vi "initialiseDevice.vi"(8 "error in (no error)":errorcluster, 10 "deviceName":string, 11 "BECHWCBasic in":refnum<class "BECHWCBasic.lvclass">) -> (0 "error out":errorcluster, 3 "BECHWCBasic out":refnum<class "BECHWCBasic.lvclass">)   [LabVIEW 2011, in "Hardware.lvlib" / "HWControllers.lvlib" / "BECHWCBasic.lvclass"]
doc: "Initialise a hardware device. \nI.e. set its initial channel states etc."
uses:
  BECHWCBasic.lvclass
  BECHWCBasic.lvclass/BECHWCBasic.ctl
  Channels/VoltOutput/AnalogOutput.lvclass
  Channels/Digital/DigitalOutput.lvclass
  HWController.lvclass
  Tools/DatabaseHelpers/DbConnection/DeviceDataBase/deviceDataBase.lvclass
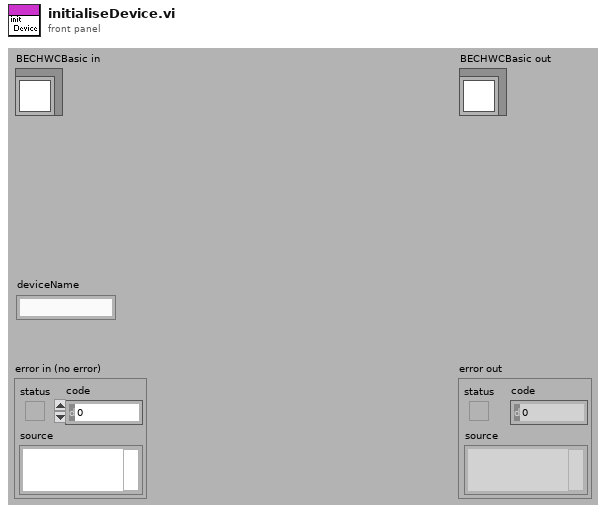
[diagram p1: front panel]
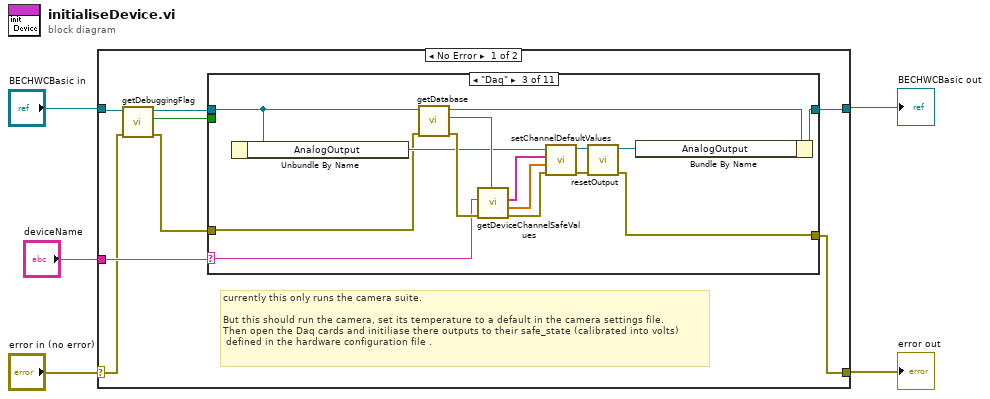
[diagram p0: block diagram]
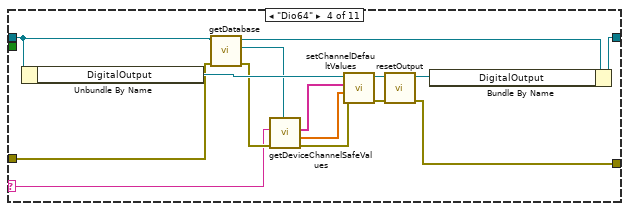
[diagram p4: hidden frame]
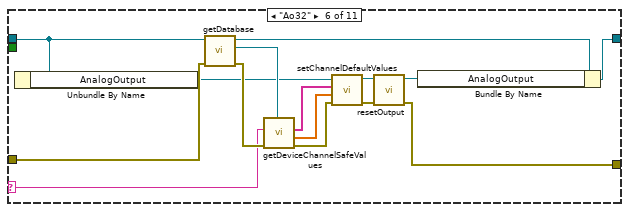
[diagram p6: hidden frame]
diagram:
  n1 = case shown="No Error" "error in (no error)" {
    selector: "error in (no error)" -> [w8 w76]
    tunnel: [w11 w76] -> w4
    tunnel: [w13 w75] -> w2
    tunnel: "BECHWCBasic in" -> [w10 w75]
    tunnel: "deviceName" -> [w12 _]
    frame No Error {
      # "currently this only runs the camera suite. \n\nBut this should run the camera, set its temperature to a default in the camera settings file.\nThen open the Daq cards and initiliase there outputs to their safe_state (calibrated into volts)\n defined in the hardware configuration file ."
      n2 = call "getDebuggingFlag.vi"("error in (no error)"=w8, "HWController.lvclass in"=w10) -> ("error out"=w7:errorcluster, "debuggingFlag"=w6:bool, "HWController.lvclass out"=w9:refnum<class "BECHWCBasic.lvclass">)  [unwired: 7 in]
      n3 = case shown="\"Daq\"" w12 {
        selector: w12 -> [_ _ w18 w37 _ w62 _ _ _ _ _]
        tunnel: w9 -> [w15 w17 w22 w41 w48 w55 w66 w68 w70 w72 w74]
        tunnel: [w15 w17 w19 w43 w48 w50 w66 w68 w70 w72 w74] -> w13
        tunnel: w7 -> [w14 w16 w21 w33 w49 w61 w65 w67 w69 w71 w73]
        tunnel: [w14 w16 w20 w42 w49 w53 w65 w67 w69 w71 w73] -> w11
        tunnel: w6 -> [_ _ _ _ _ _ _ _ _ _ _]
        frame "No Hardware", Default {
        }
        frame "UsbDAQ" {
        }
        frame "Daq" {
          n4 = Unbundle By Name(w22) -> ("AnalogOutput"=w25:refnum<class "AnalogOutput.lvclass">)
          n5 = call "getDatabase.vi"("error in (no error)"=w21, "HWController in"=w22) -> ("error out"=w31:errorcluster, "deviceDataBase"=w32:refnum<class "deviceDataBase.lvclass">, "HWController out"=w23:refnum<class "BECHWCBasic.lvclass">)  [unwired: 7 in]
          n6 = call "getDeviceChannelSafeValues.vi"("error in (no error)"=w31, "device_name"=w18, "deviceDataBase in"=w32) -> ("error out"=w30:errorcluster, "SafeVaues"=w29:dbl[], "ChannelAddresses"=w28:string[])  [unwired: 5 in, 1 out]
          n7 = call "setChannelDefaultValues.vi"("error in (no error)"=w30, "calibratedValues"=w29, "channel_addresses"=w28, "AnalogOutput in"=w25) -> ("error out"=w26:errorcluster, "AnalogOutput out"=w27:refnum<class "AnalogOutput.lvclass">)  [unwired: 6 in]
          n8 = call-dynamic "resetOutput.vi"("error in (no error)"=w26, "AnalogOutput in"=w27) -> ("error out"=w20:errorcluster, "AnalogOutput out"=w24:refnum<class "AnalogOutput.lvclass">)  [unwired: 8 in]
          n9 = Bundle By Name(cluster=w23, "AnalogOutput"=w24) -> (w19:refnum<class "BECHWCBasic.lvclass">)
        }
        frame "Dio64" {
          n10 = Unbundle By Name(w41) -> ("DigitalOutput"=w47:refnum<class "DigitalOutput.lvclass">)
          n11 = call "getDatabase.vi"("error in (no error)"=w33, "HWController in"=w41) -> ("error out"=w38:errorcluster, "deviceDataBase"=w39:refnum<class "deviceDataBase.lvclass">, "HWController out"=w40:refnum<class "BECHWCBasic.lvclass">)  [unwired: 7 in]
          n12 = call "getDeviceChannelSafeValues.vi"("error in (no error)"=w38, "device_name"=w37, "deviceDataBase in"=w39) -> ("error out"=w34:errorcluster, "SafeVaues"=w35:dbl[], "ChannelAddresses"=w36:string[])  [unwired: 5 in, 1 out]
          n13 = call-dynamic "setChannelDefaultValues.vi"("error in (no error)"=w34, "calibratedValues"=w35, "channel_addresses"=w36, "DigitalOutput in"=w47) -> ("error out"=w45:errorcluster, "DigitalOutput out"=w46:refnum<class "DigitalOutput.lvclass">)  [unwired: 6 in]
          n14 = call-dynamic "resetOutput.vi"("error in (no error)"=w45, "DigitalOutput in"=w46) -> ("error out"=w42:errorcluster, "DigitalOutput out"=w44:refnum<class "DigitalOutput.lvclass">)  [unwired: 8 in]
          n15 = Bundle By Name(cluster=w40, "DigitalOutput"=w44) -> (w43:refnum<class "BECHWCBasic.lvclass">)
        }
        frame "Ao8" {
        }
        frame "Ao32" {
          n16 = Unbundle By Name(w55) -> ("AnalogOutput"=w54:refnum<class "AnalogOutput.lvclass">)
          n17 = call "getDatabase.vi"("error in (no error)"=w61, "HWController in"=w55) -> ("error out"=w63:errorcluster, "deviceDataBase"=w64:refnum<class "deviceDataBase.lvclass">, "HWController out"=w51:refnum<class "BECHWCBasic.lvclass">)  [unwired: 7 in]
          n18 = call "getDeviceChannelSafeValues.vi"("error in (no error)"=w63, "device_name"=w62, "deviceDataBase in"=w64) -> ("error out"=w60:errorcluster, "SafeVaues"=w59:dbl[], "ChannelAddresses"=w58:string[])  [unwired: 5 in, 1 out]
          n19 = call "setChannelDefaultValues.vi"("error in (no error)"=w60, "calibratedValues"=w59, "channel_addresses"=w58, "AnalogOutput in"=w54) -> ("error out"=w56:errorcluster, "AnalogOutput out"=w57:refnum<class "AnalogOutput.lvclass">)  [unwired: 6 in]
          n20 = call-dynamic "resetOutput.vi"("error in (no error)"=w56, "AnalogOutput in"=w57) -> ("error out"=w53:errorcluster, "AnalogOutput out"=w52:refnum<class "AnalogOutput.lvclass">)  [unwired: 8 in]
          n21 = Bundle By Name(cluster=w51, "AnalogOutput"=w52) -> (w50:refnum<class "BECHWCBasic.lvclass">)
        }
        frame "ArbWave" {
        }
        frame "ICCamera" {
        }
        frame "AndorIKon" {
        }
        frame "S1010" {
        }
        frame "C100" {
        }
      }
    }
    frame Error {
    }
  }
  "error out" <- w4
  "BECHWCBasic out" <- w2
